vi "Configure Protect RMS UVP.vi"(8 "error in":errorcluster, 9 "Level(V)":dbl min=0.0, 10 "Phase":enum16{"A", "B", "C", "ALL"}(ring), 11 "VISA resource name":refnum<visa-resource-name>) -> (0 "error out":errorcluster, 3 "VISA resource name out":refnum<visa-resource-name>)   [LabVIEW 2020, in "IT-M7700.lvlib"]
doc: "The UVP(RMS) command is used to set the UVP(RMS) of a power supply.\n<b>Phase</b>\n0: A\n1: B\n2: C\n3: ALL\n<b>Level(V)</b>\n0-MAX"
uses:
  <instrlib>/IT-M7700/IT-M7700.lvlib
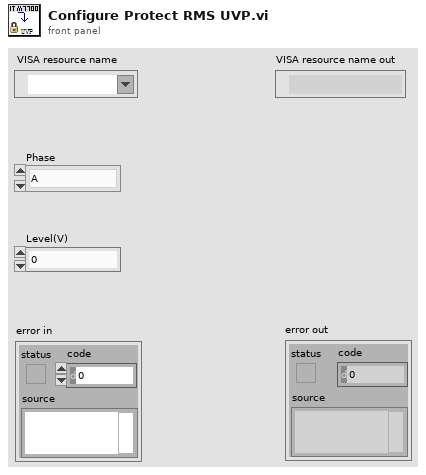
[diagram p1: front panel]
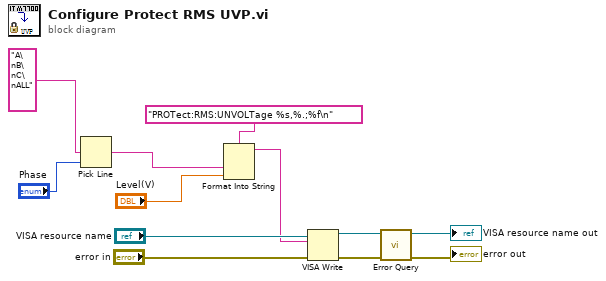
[diagram p0: block diagram]
diagram:
  n1 = Pick Line(multi-line string="A\nB\nC\nALL" ("多行字符串"), line index="Phase") -> (output string=w4:string)  [unwired: 1 in]
  n2 = Format Into String(format string="PROTect:RMS:UNVOLTage %s,%.;%f\n", w4, "Level(V)") -> (resulting string=w9:string)  [unwired: 2 in, 1 out]
  n3 = VISA Write(VISA resource name="VISA resource name", write buffer=w9, error in (no error)="error in") -> (VISA resource name out=w8:refnum<visa-resource-name>, error out=w7:errorcluster)  [unwired: 1 out]
  n4 = call <instrlib>:"Error Query.vi"("error in"=w7, "VISA resource name"=w8) -> ("error out"=→"error out":errorcluster, "VISA resource name out"=→"VISA resource name out":refnum<visa-resource-name>)  [unwired: 6 in, 2 out]
